vi "短日期时间转长日期格式.vi"(10 "table输入":string(combo), 11 "data":string[][](table)) -> (3 "输出数组":string[][](array[string]))   [LabVIEW 2016, in "数据传输系统-04.lvlib"]
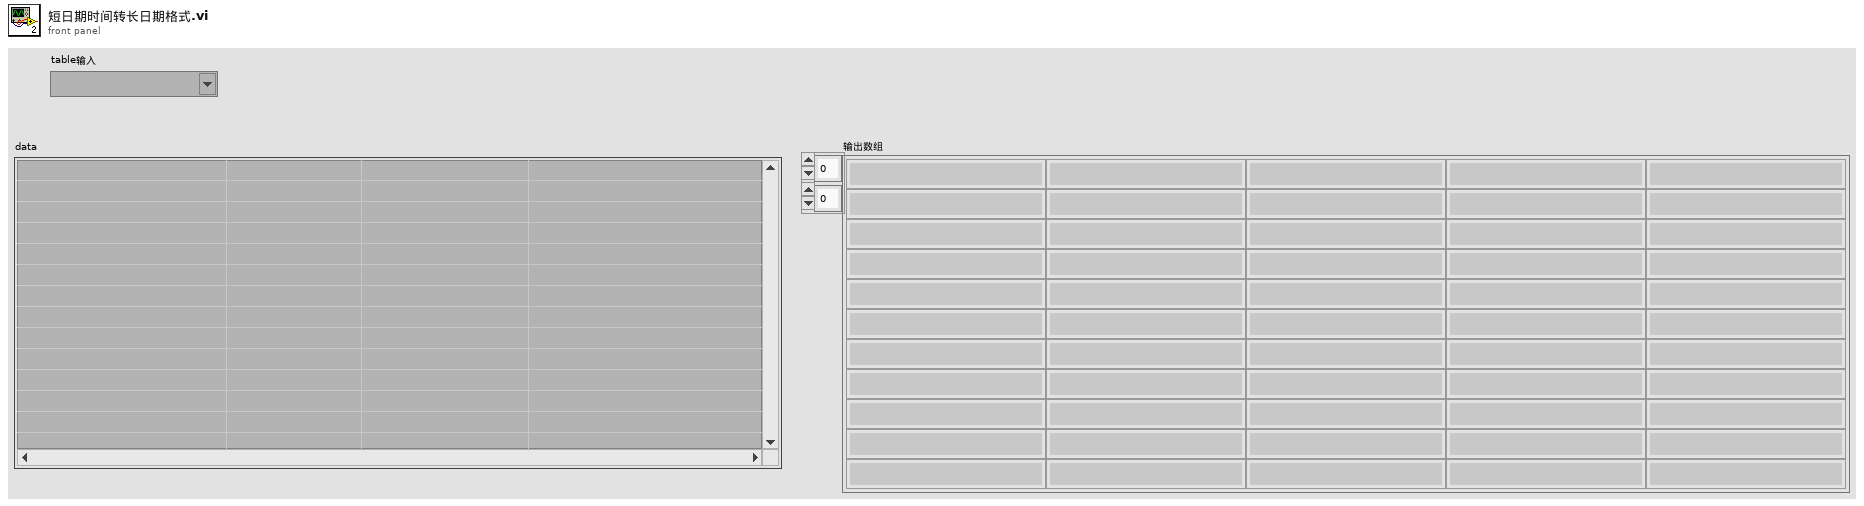
[diagram p1: front panel]
types:
  T1 = typedef "LVDateTimeRec.ctl" = cluster{"秒数的小数部分":dbl, "秒":i32, "分":i32, "时":i32, "日":i32, "月":i32, "年":i32, "天数（周）":i32, "天数（年）":i32, "DST":i32}
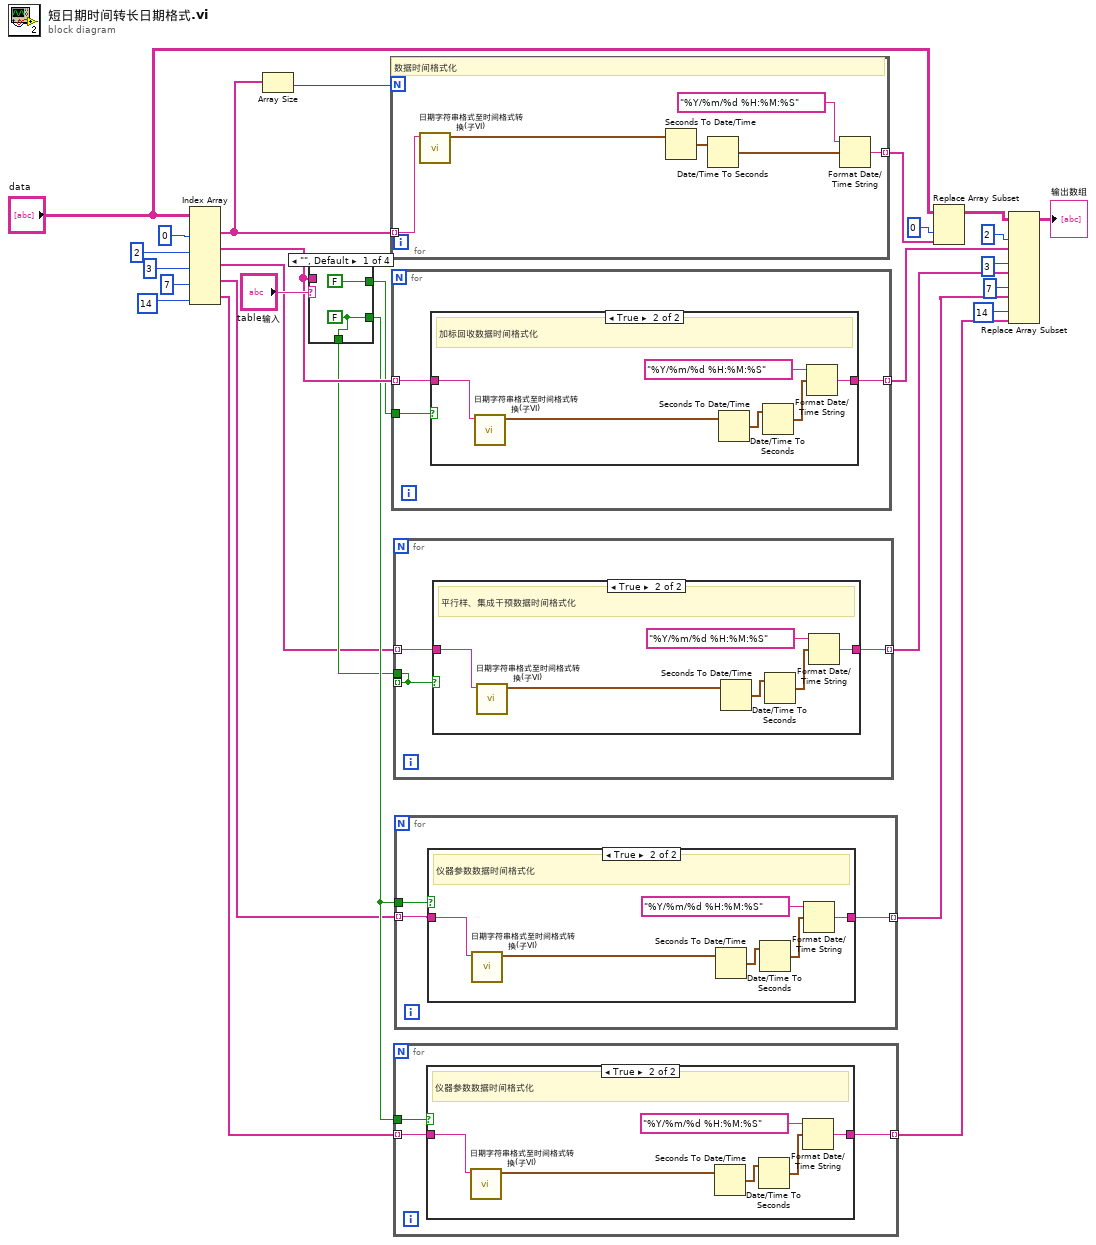
[diagram p0: block diagram]
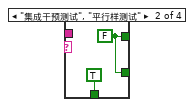
[diagram p6: hidden frame]
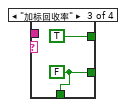
[diagram p7: hidden frame]
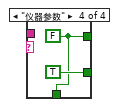
[diagram p8: hidden frame]
diagram:
  n1 = Index Array(array="data", index (col) #1=0 ("禁用的索引 (列)"), index (col) #2=2 ("索引 (列)"), index (col) #3=3 ("索引 (列)"), index (col) #4=7 ("索引 (列)"), index (col) #5=14 ("索引 (列)")) -> (element #1=w20:string[], element #2=w18:string[], element #3=w8:string[], element #4=w13:string[], element #5=w14:string[])  [unwired: 5 in]
  n2 = Array Size(array=w20) -> (size(s)=w19:i32)
  n3 = case shown="\"\", Default" "table输入" {
    tunnel: [FALSE w31 TRUE w35] -> w17
    tunnel: w18 -> [_ _ _ _]
    tunnel: [w29 w31 w33 TRUE] -> w15
    tunnel: [w29 TRUE w33 w35] -> w9
    frame "", Default {
      w29 = FALSE
    }
    frame "集成干预测试", "平行样测试" {
      w31 = FALSE
    }
    frame "加标回收率" {
      w33 = FALSE
    }
    frame "仪器参数" {
      w35 = FALSE
    }
  }
  n4 = for {
    N: w19 -> [_]
    tunnel: [w38] -> w24 mode=indexing
    tunnel: w20 -> [w37] mode=indexing
    # "数据时间格式化"
    n5 = call "日期字符串格式至时间格式转换(子VI).vi"("data[0]"=w37) -> ("time stamp"=w41:timestamp)  [unwired: 10 in]
    n6 = Seconds To Date/Time(time stamp (now)=w41) -> (date time rec=w42:T1)  [unwired: 1 in]
    n7 = Date/Time To Seconds(2:w42) -> (0:w40:timestamp)  [unwired: 1 in]
    n8 = Format Date/Time String(time format string (%c)="%Y/%m/%d %H:%M:%S" ("时间格式字符串(%c)"), seconds (now)=w40) -> (date/time string=w38:string)  [unwired: 1 in]
  }
  n9 = for {
    tunnel: w18 -> [w45] mode=indexing
    tunnel: w17 -> [w44]
    tunnel: [w43] -> w16 mode=indexing
    n10 = case shown="True" w44 {
      tunnel: [w46 w48] -> w43
      tunnel: w45 -> [w46 w47]
      frame False {
      }
      frame True {
        # "加标回收数据时间格式化"
        n11 = call "日期字符串格式至时间格式转换(子VI).vi"("data[0]"=w47) -> ("time stamp"=w50:timestamp)  [unwired: 10 in]
        n12 = Seconds To Date/Time(time stamp (now)=w50) -> (date time rec=w49:T1)  [unwired: 1 in]
        n13 = Date/Time To Seconds(2:w49) -> (0:w51:timestamp)  [unwired: 1 in]
        n14 = Format Date/Time String(time format string (%c)="%Y/%m/%d %H:%M:%S" ("时间格式字符串(%c)"), seconds (now)=w51) -> (date/time string=w48:string)  [unwired: 1 in]
      }
    }
  }
  n15 = for {
    tunnel: w8 -> [w55] mode=indexing
    tunnel: [w53] -> _ mode=indexing
    tunnel: [w54] -> w4 mode=indexing
    tunnel: w9 -> [w53]
    n16 = case shown="True" w53 {
      tunnel: [w56 w58] -> w54
      tunnel: w55 -> [w56 w57]
      frame False {
      }
      frame True {
        # "平行样、集成干预数据时间格式化"
        n17 = call "日期字符串格式至时间格式转换(子VI).vi"("data[0]"=w57) -> ("time stamp"=w60:timestamp)  [unwired: 10 in]
        n18 = Seconds To Date/Time(time stamp (now)=w60) -> (date time rec=w59:T1)  [unwired: 1 in]
        n19 = Date/Time To Seconds(2:w59) -> (0:w61:timestamp)  [unwired: 1 in]
        n20 = Format Date/Time String(time format string (%c)="%Y/%m/%d %H:%M:%S" ("时间格式字符串(%c)"), seconds (now)=w61) -> (date/time string=w58:string)  [unwired: 1 in]
      }
    }
  }
  n21 = for {
    tunnel: w14 -> [w65] mode=indexing
    tunnel: w15 -> [w64]
    tunnel: [w63] -> w3 mode=indexing
    n22 = case shown="True" w64 {
      tunnel: [w66 w68] -> w63
      tunnel: w65 -> [w66 w67]
      frame False {
      }
      frame True {
        # "仪器参数数据时间格式化"
        n23 = call "日期字符串格式至时间格式转换(子VI).vi"("data[0]"=w67) -> ("time stamp"=w70:timestamp)  [unwired: 10 in]
        n24 = Seconds To Date/Time(time stamp (now)=w70) -> (date time rec=w69:T1)  [unwired: 1 in]
        n25 = Date/Time To Seconds(2:w69) -> (0:w71:timestamp)  [unwired: 1 in]
        n26 = Format Date/Time String(time format string (%c)="%Y/%m/%d %H:%M:%S" ("时间格式字符串(%c)"), seconds (now)=w71) -> (date/time string=w68:string)  [unwired: 1 in]
      }
    }
  }
  n27 = for {
    tunnel: w13 -> [w75] mode=indexing
    tunnel: [w74] -> w2 mode=indexing
    tunnel: w15 -> [w73]
    n28 = case shown="True" w73 {
      tunnel: [w76 w78] -> w74
      tunnel: w75 -> [w76 w77]
      frame False {
      }
      frame True {
        # "仪器参数数据时间格式化"
        n29 = call "日期字符串格式至时间格式转换(子VI).vi"("data[0]"=w77) -> ("time stamp"=w80:timestamp)  [unwired: 10 in]
        n30 = Seconds To Date/Time(time stamp (now)=w80) -> (date time rec=w79:T1)  [unwired: 1 in]
        n31 = Date/Time To Seconds(2:w79) -> (0:w81:timestamp)  [unwired: 1 in]
        n32 = Format Date/Time String(time format string (%c)="%Y/%m/%d %H:%M:%S" ("时间格式字符串(%c)"), seconds (now)=w81) -> (date/time string=w78:string)  [unwired: 1 in]
      }
    }
  }
  n33 = Replace Array Subset(array="data", new element=w24, index (col)=0 ("禁用的索引 (列)")) -> (w22:string[][])  [unwired: 1 in]
  n34 = Replace Array Subset(array=w22, new element #1=w16, index (col) #1=2 ("索引 (列)"), new element #2=w4, index (col) #2=3 ("索引 (列)"), new element #3=w2, index (col) #3=7 ("索引 (列)"), new element #4=w3, index (col) #4=14 ("索引 (列)")) -> (→"输出数组":string[][])  [unwired: 4 in]
